vi "Stop All Actors.vi"(8 "error in (no error)":errorcluster, 11 "input cluster":T1) -> (0 "error out":errorcluster)   [LabVIEW 2020, in "Supervisor.lvlib" / "Supervisor.lvclass"]
uses:
  Supervisor.lvclass
  Supervisor.lvclass/Supervisor.ctl
  <vilib>/ActorFramework/Stop Msg/Stop Msg.lvclass
  DAQ DI/DAQ DI Messages/Crear DAQ Task Msg/Crear DAQ Task Msg.lvclass
  DAQ AI/DAQ AI Messages/Crear DAQ Task Msg/Crear DAQ Task Msg.lvclass
  <vilib>/ActorFramework/Message Enqueuer/Message Enqueuer.lvclass
  TypeDef/Actor Queues.ctl
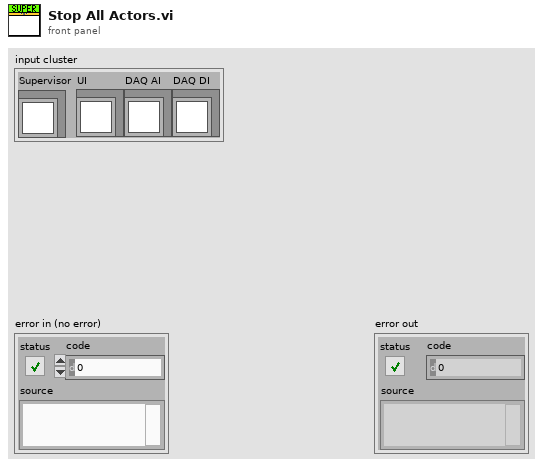
[diagram p1: front panel]
types:
  T1 = typedef "Supervisor.lvlib/Supervisor.lvclass/Actor Queues.ctl" = cluster{"Supervisor":refnum<class "Message Enqueuer.lvclass">, "UI":refnum<class "Message Enqueuer.lvclass">, "DAQ AI":refnum<class "Message Enqueuer.lvclass">, "DAQ DI":refnum<class "Message Enqueuer.lvclass">}
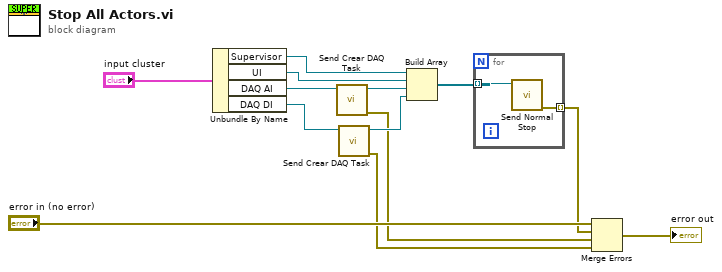
[diagram p0: block diagram]
diagram:
  n1 = Unbundle By Name("input cluster") -> ("Supervisor"=w13:refnum<class "Message Enqueuer.lvclass">, "UI"=w12:refnum<class "Message Enqueuer.lvclass">, "DAQ AI"=w9:refnum<class "Message Enqueuer.lvclass">, "DAQ DI"=w8:refnum<class "Message Enqueuer.lvclass">)
  n2 = call "Send Crear DAQ Task.vi"("Message Enqueuer"=w9) -> ("error out"=w3:errorcluster, "Message Enqueuer out"=w6:refnum<class "Message Enqueuer.lvclass">)  [unwired: 9 in]
  n3 = call "Send Crear DAQ Task.vi"("Message Enqueuer"=w8) -> ("error out"=w2:errorcluster, "Message Enqueuer out"=w7:refnum<class "Message Enqueuer.lvclass">)  [unwired: 9 in]
  n4 = Build Array(w13, w12, w6, w7) -> (w11:refnum<class "Message Enqueuer.lvclass">[])
  n5 = for {
    tunnel: w11 -> [w15] mode=indexing
    tunnel: [w14] -> w4 mode=indexing
    n6 = call <vilib>:"Send Normal Stop.vi"("Message Enqueuer"=w15) -> ("error out"=w14:errorcluster)  [unwired: 10 in]
  }
  n7 = Merge Errors("error in (no error)", w4, w3, w2) -> (→"error out":errorcluster)
